vi "dfd_DA Load Input.vi"(10 "load":bool, 11 "x":fxp<+/-,15,1> format="%.15g") -> (3 "bit array in":bool[](array[boolean]))   [LabVIEW 2017]
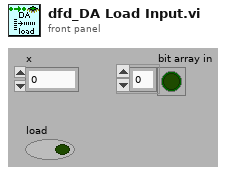
[diagram p1: front panel]
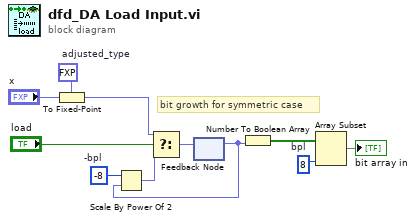
[diagram p0: block diagram]
diagram:
  w1 = 8  # bpl
  w5 = fxp<+/-,32,16> 0.0  # adjusted_type
  w9 = -8  # -bpl
  # "bit growth for symmetric case"
  n1 = To Fixed-Point(fixed-point type=w5, number="x") -> (fixed-point=w4:fxp<+/-,32,16>)
  n2 = feedback #1() -> (w6:fxp<+/-,32,16>)  [unwired: 1 out]
  n3 = Scale By Power Of 2(n=w9, x=w6) -> (x*2^n=w8:fxp<+/-,32,16>)
  n4 = Select(t=w4, s="load", f=w8) -> (s? t:f=w7:fxp<+/-,32,16>)
  n5 = feedback-in #1(w7) -> ()
  n6 = Number To Boolean Array(number=w6) -> (Boolean array=w2:bool[])
  n7 = Array Subset(array=w2, length=w1) -> (→"bit array in":bool[])  [unwired: 1 in]
